vi "Measurement UI.vi"() -> ()   [LabVIEW 2025, in "I2C Bus Monitor UI.lvlib"]
uses:
  I2C Bus Monitor UI.lvlib
  OOB gRPC Client/RPC Messages/hwval_GenericRequest.ctl
  SubVIs/Save CSV.vi
  SubVIs/Table Buffer - Create.vi
  SubVIs/Table Buffer - Destroy.vi
  OOB gRPC Client/OOB gRPC Client.lvlib
panel:
  out "RUNNING":bool
  in  "Monitor Tab":enum32{"Monitor", "Scan"}(tab)
  out "# TXNS IN TABLE":i32
  in  "PauseResume":bool=TRUE
  out "STREAMING":bool
  in  "CSV FILE PATH":path
  in  "Save CSV":bool
  out "# TXNS IN BUFFER":i32
  in  "Clear":bool
  out "MONITOR TABLE":string[][](table)
  in  "Scan Bus":bool
  out "Scan Table":string[][](table)
  out "BUSY":bool
  in  "Debug&Hidden":enum32{"Debug", "Hidden"}(tab)
  out "Message Buffer Pressure (Logic)":i32
  out "Transactions in Buffer (UI)":i32
  out "FIFO Overflow":bool
  out "FIFO Pressure":u32
  out "Measurement Logic Counter":i32
  out "FIFO Msg Fetch Count":i32
  out "OOB gRPC Port":i32
  in  "Bitfile Path":string
  in  "Alias Name":string
  in  "Serial Input":string
  out "Error (Logic)":string
  out "Scanned Addresses":i32[](array[numeric]) format="%.0x"
  out "Status":string
  in  "Send I2C CMD":bool
  in  "R/W":bool
  in  "DATA":u8 format="%02x"
  in  "REG. ADDR.":u16 format="%04x"
  in  "SLAVE ADDR.":u8 format="%02x"
  in  "Send I2C Script":bool
  in  "SCRIPT FILE PATH":path
  in  "SERIAL INPUT (SI)":u32(ring)
  in  "RESOURCE NAME":u32(ring)
  # "NOTE:\nFlat Box sizes are specifically chosen to fit into IS small panel without a horizontal scrollbar"
  # "CONFIGURATION"
  # "I2C TRANSACTIONS"
  # "I2C MONITOR"
  # "STATUS"
  # "These controls are mainly used to transfer data from logic to ui via configs/results, but don't need to be visible."
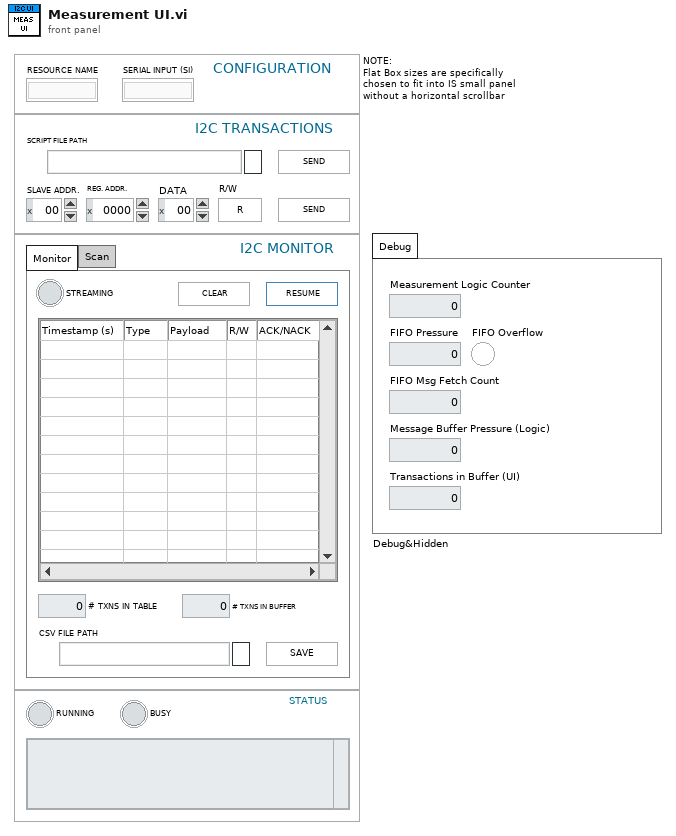
[diagram p1: front panel]
types:
  T1 = cluster{"Measurement Logic Counter":refnum<vi>, "OOB gRPC Port":refnum<vi>, "Bitfile Path":refnum<vi>, "RESOURCE NAME":refnum<vi>, "Alias Name":refnum<vi>, "SERIAL INPUT (SI)":refnum<vi>, "Serial Input":refnum<vi>, "MONITOR TABLE":refnum<vi>, "FIFO Msg Fetch Count":refnum<vi>, "STREAMING":refnum<vi>, "PauseResume":refnum<vi>, "Transactions in Buffer (UI)":refnum<vi>, "CSV FILE PATH":refnum<vi>, "BUSY":refnum<vi>, "Status":refnum<vi>, "Error (Logic)":refnum<vi>, "Scan Table":refnum<vi>, "Scanned Addresses":refnum<vi>, "# TXNS IN BUFFER":refnum<vi>, "# TXNS IN TABLE":refnum<vi>, "RUNNING":refnum<vi>}
  T2 = typedef "OOB gRPC Client.lvlib/hwval_GenericRequest.ctl" = cluster{"Command":string, "Payload":u8[]}
  T3 = typedef "OOB gRPC Client.lvlib/hwval_GenericResponse.ctl" = cluster{"Payload":u8[]}
  T4 = typedef "grpc-lvsupport-release.lvlib/grpcId.ctl" = u64
  T5 = cluster{"NewVal":bool, "SLAVE ADDR.":u8, "REG. ADDR.":u16, "DATA":u8, "R/W":bool}
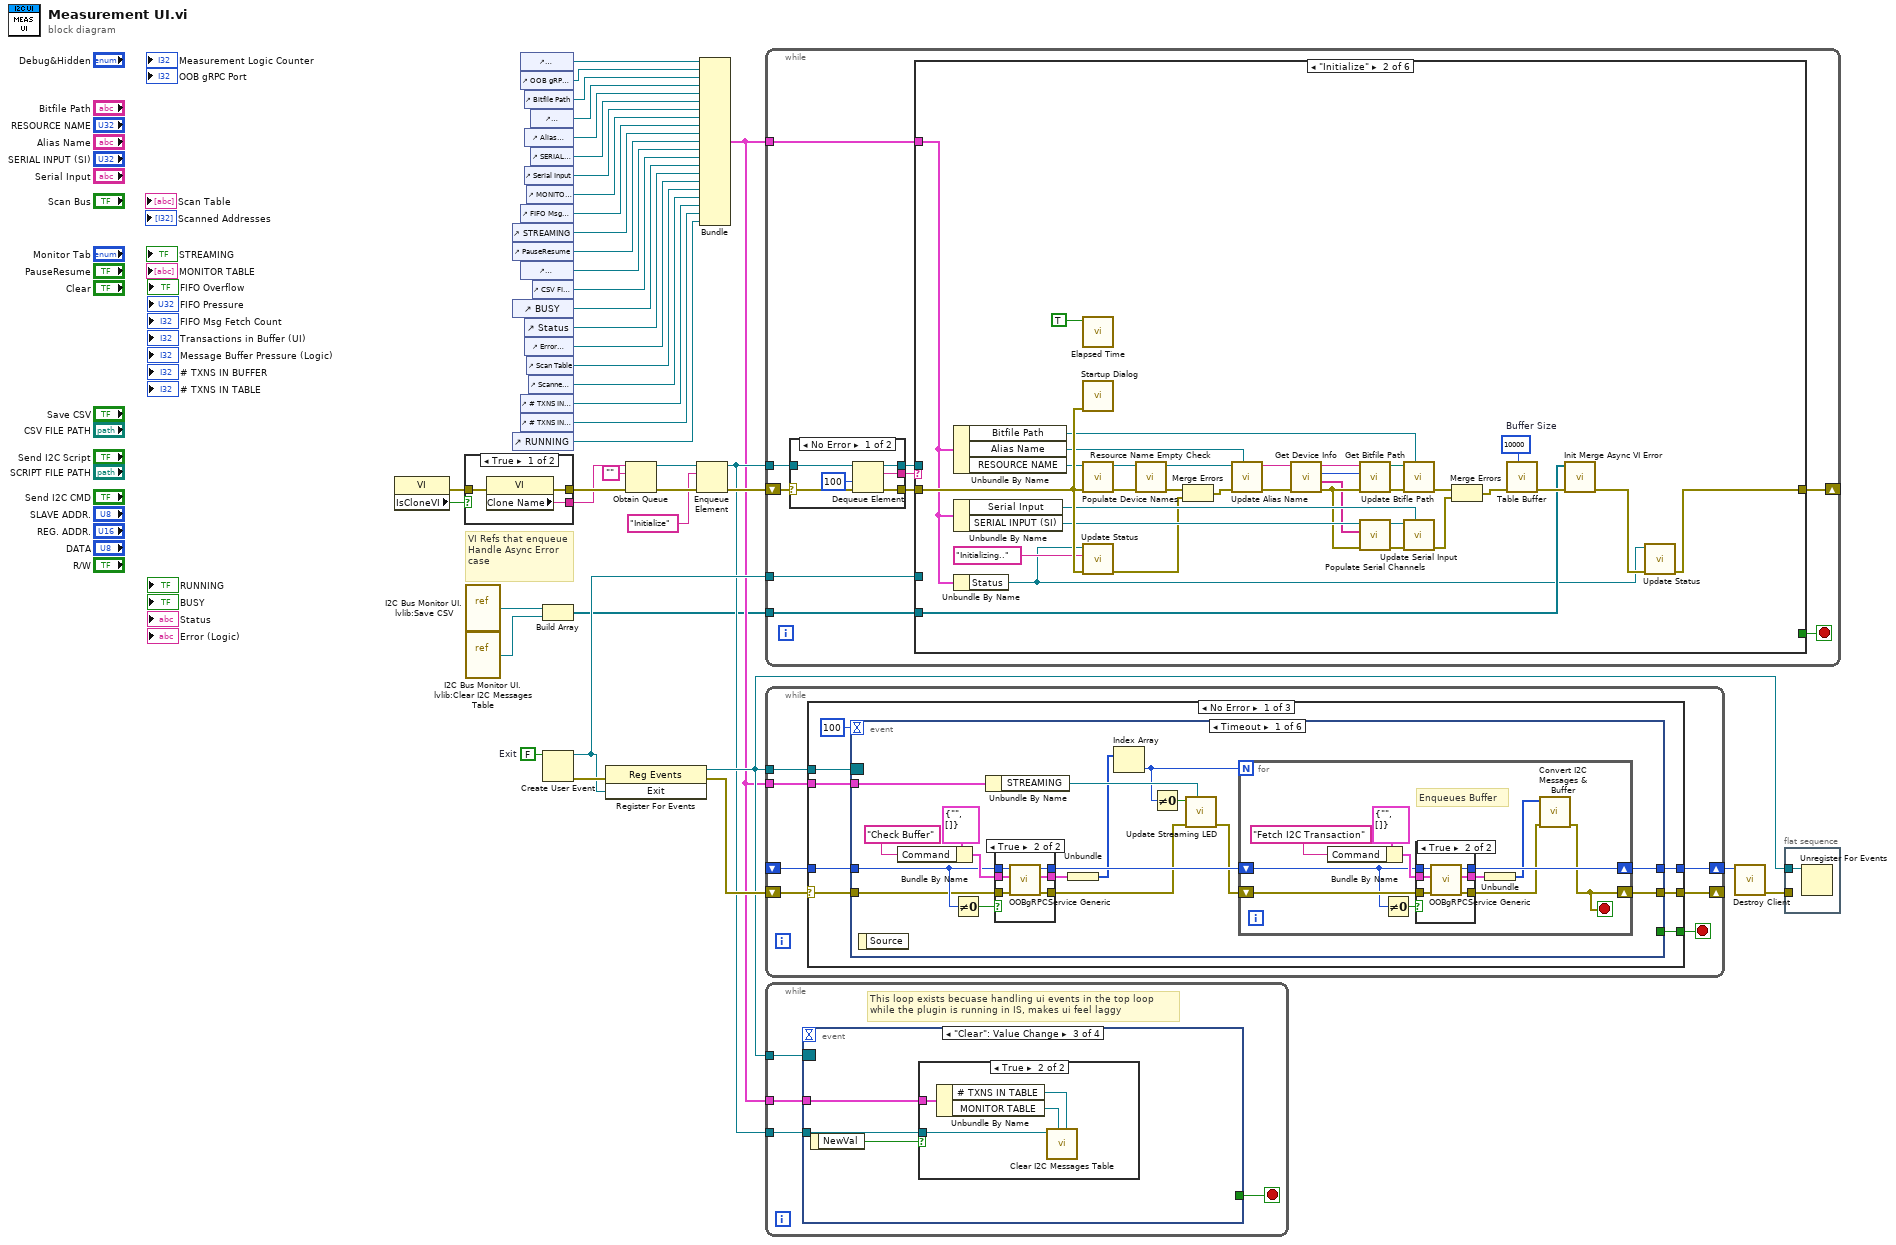
[diagram p0: block diagram]
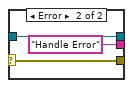
[diagram p2: hidden frame]
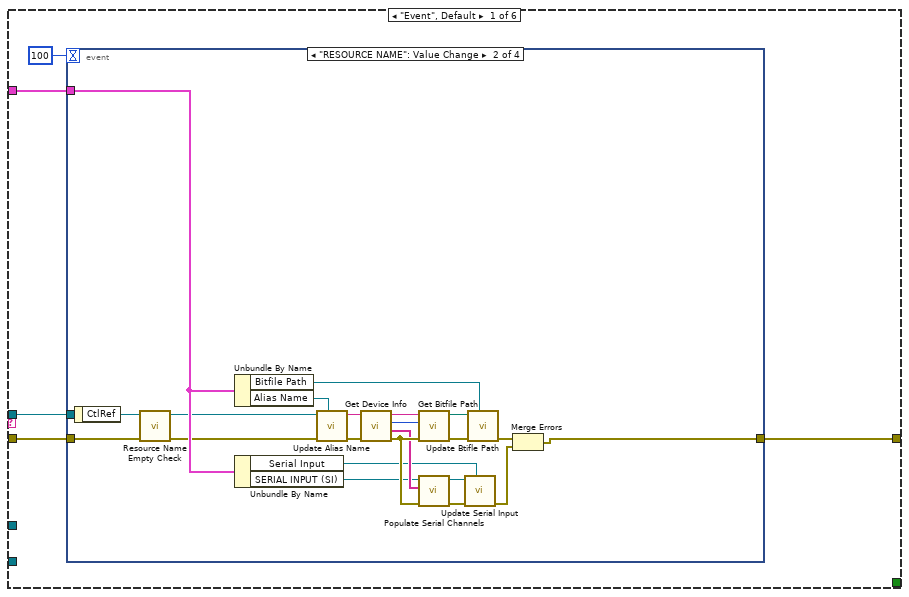
[diagram p3: hidden frame]
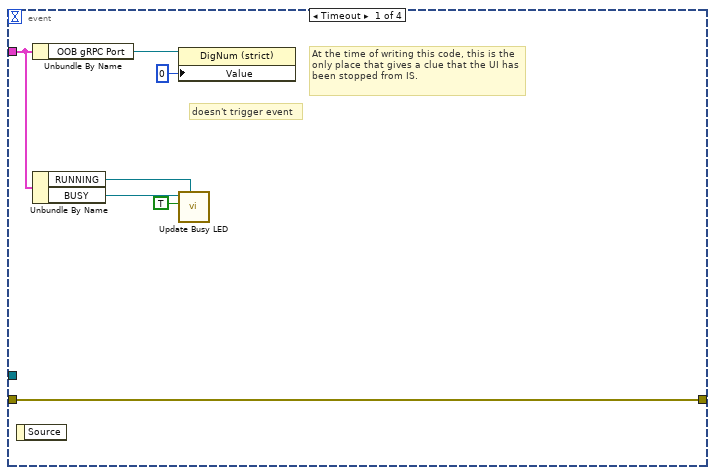
[diagram p4: hidden frame]
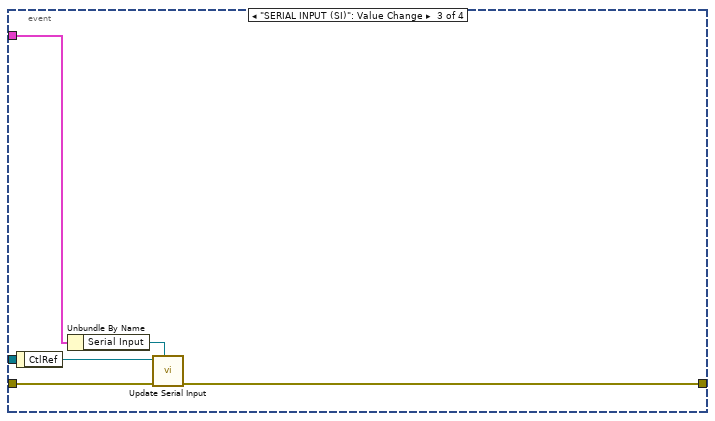
[diagram p5: hidden frame]
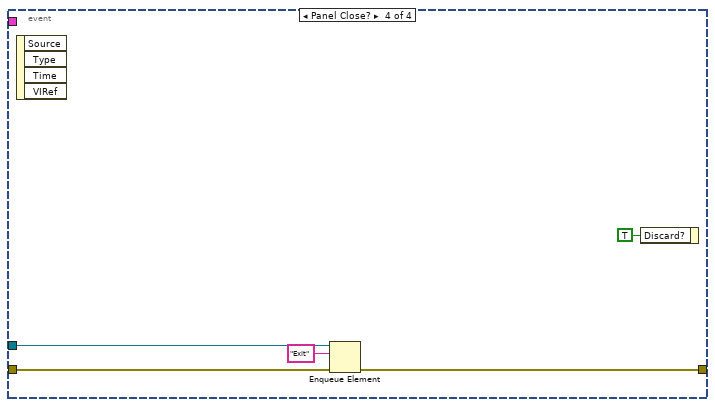
[diagram p6: hidden frame]
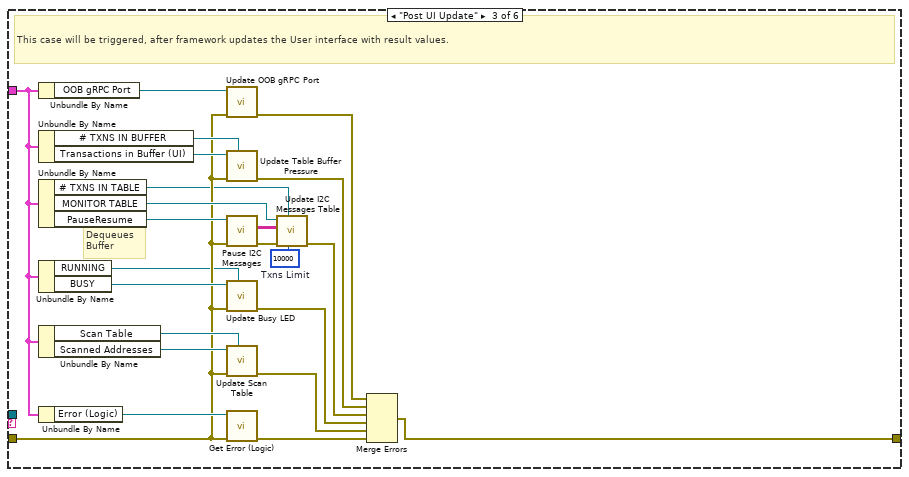
[diagram p7: hidden frame]
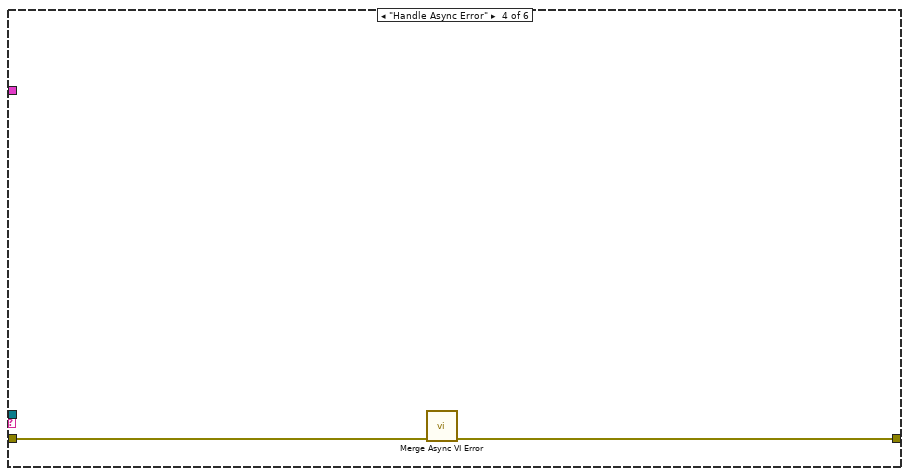
[diagram p8: hidden frame]
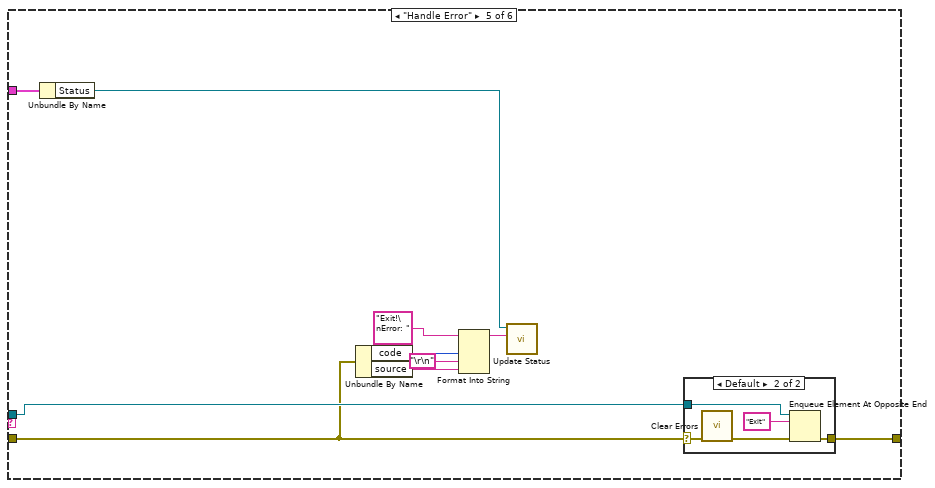
[diagram p9: hidden frame]
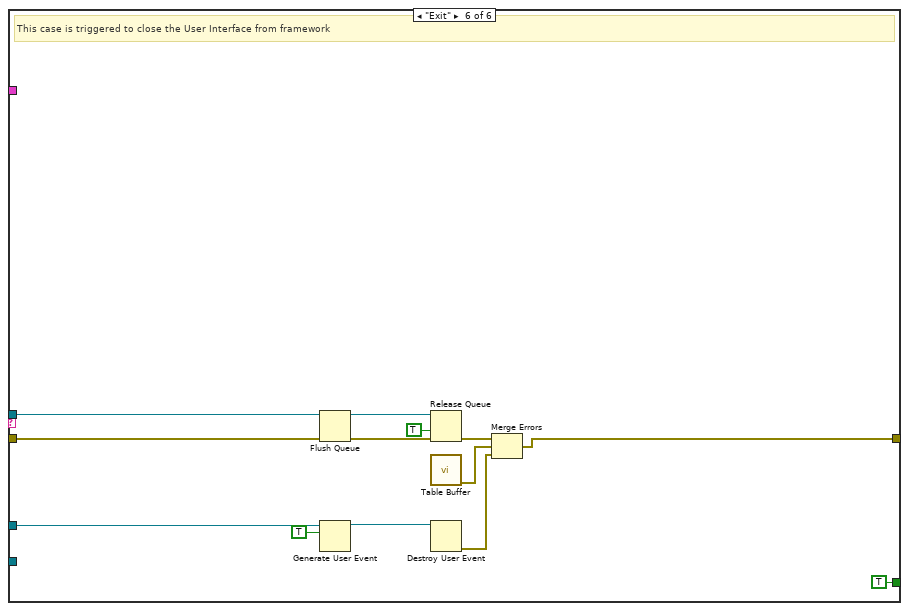
[diagram p11: hidden frame]
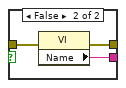
[diagram p12: hidden frame]
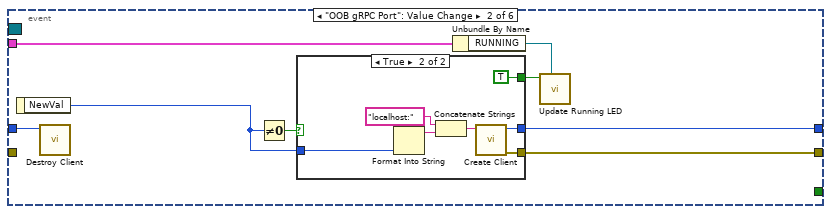
[diagram p15: hidden frame]
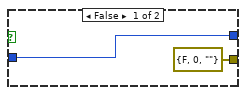
[diagram p16: hidden frame]
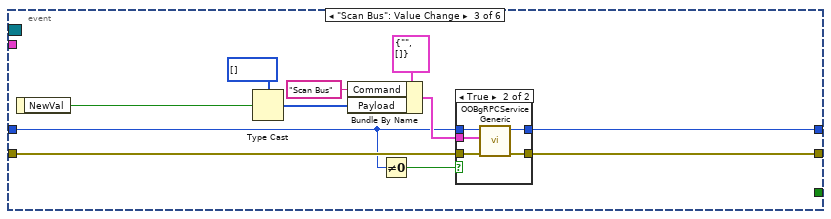
[diagram p17: hidden frame]
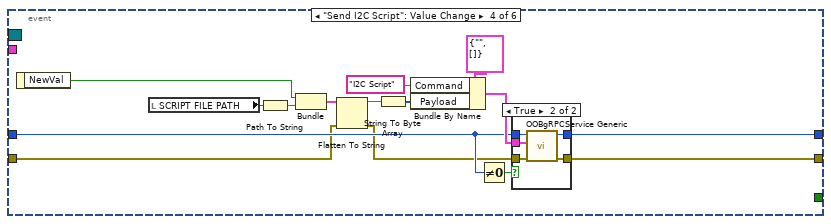
[diagram p19: hidden frame]
diagram:
  w33 = FALSE  # Exit
  # "VI Refs that enqueue Handle Async Error case"
  n1 = property class="VI"() -> (error out=w29:errorcluster, "IsCloneVI"=w34:bool)  [unwired: 2 in, 1 out]
  n2 = case shown="True" w34 {
    tunnel: [w45 w48] -> w41
    tunnel: [w44 w47] -> w40
    tunnel: w29 -> [w43 w46]
    frame True {
      n3 = property class="VI"(error in=w43) -> (error out=w45:errorcluster, "Clone Name"=w44:string)  [unwired: 1 in, 1 out]
    }
    frame False {
      n4 = property class="VI"(error in=w46) -> (error out=w48:errorcluster, "Name"=w47:string)  [unwired: 1 in, 1 out]
    }
  }
  n5 = vi-ref "I2C Bus Monitor UI.lvlib:Save CSV.vi"() -> (w9:refnum<vi>)
  n6 = vi-ref "I2C Bus Monitor UI.lvlib:Clear I2C Messages Table.vi"() -> (w4:refnum<vi>)
  n7 = control-ref of="STREAMING"() -> (w15:refnum<vi>)
  n8 = control-ref of="PauseResume"() -> (w21:refnum<vi>)
  n9 = control-ref of="BUSY"() -> (w13:refnum<vi>)
  n10 = control-ref of="RUNNING"() -> (w1:refnum<vi>)
  n11 = control-ref of="Measurement Logic Counter"() -> (w14:refnum<vi>)
  n12 = control-ref of="OOB gRPC Port"() -> (w27:refnum<vi>)
  n13 = control-ref of="FIFO Msg Fetch Count"() -> (w28:refnum<vi>)
  n14 = control-ref of="Transactions in Buffer (UI)"() -> (w20:refnum<vi>)
  n15 = control-ref of="# TXNS IN BUFFER"() -> (w5:refnum<vi>)
  n16 = control-ref of="# TXNS IN TABLE"() -> (w2:refnum<vi>)
  n17 = control-ref of="Bitfile Path"() -> (w22:refnum<vi>)
  n18 = control-ref of="Alias Name"() -> (w24:refnum<vi>)
  n19 = control-ref of="Serial Input"() -> (w26:refnum<vi>)
  n20 = control-ref of="Status"() -> (w11:refnum<vi>)
  n21 = control-ref of="Error (Logic)"() -> (w10:refnum<vi>)
  n22 = control-ref of="MONITOR TABLE"() -> (w18:refnum<vi>)
  n23 = control-ref of="Scan Table"() -> (w7:refnum<vi>)
  n24 = control-ref of="Scanned Addresses"() -> (w6:refnum<vi>)
  n25 = control-ref of="RESOURCE NAME"() -> (w23:refnum<vi>)
  n26 = control-ref of="SERIAL INPUT (SI)"() -> (w25:refnum<vi>)
  n27 = control-ref of="CSV FILE PATH"() -> (w19:refnum<vi>)
  n28 = Build Array(w9, w4) -> (w8:refnum<vi>[])
  n29 = Create User Event(user event datatype=w33) -> (user event=w30:refnum<user-event>, error out=w32:errorcluster)  [unwired: 1 in]
  n30 = register-events(error in=w32, w30) -> (reference out=w17:refnum<event-registration>, error out=w42:errorcluster)  [unwired: 1 in]
  n31 = Obtain Queue(name (unnamed)=w40, element data type="", error in (no error)=w41) -> (queue out=w37:refnum<queue>, error out=w39:errorcluster)  [unwired: 2 in, 1 out]
  n32 = Enqueue Element(queue=w37, element="Initialize", error in (no error)=w39) -> (queue out=w16:refnum<queue>, error out=w38:errorcluster)  [unwired: 1 in, 1 out]
  n33 = Bundle("Measurement Logic Counter"=w14, "OOB gRPC Port"=w27, "Bitfile Path"=w22, "RESOURCE NAME"=w23, "Alias Name"=w24, "SERIAL INPUT (SI)"=w25, "Serial Input"=w26, "MONITOR TABLE"=w18, "FIFO Msg Fetch Count"=w28, "STREAMING"=w15, "PauseResume"=w21, "Transactions in Buffer (UI)"=w20, "CSV FILE PATH"=w19, "BUSY"=w13, "Status"=w11, "Error (Logic)"=w10, "Scan Table"=w7, "Scanned Addresses"=w6, "# TXNS IN BUFFER"=w5, "# TXNS IN TABLE"=w2, "RUNNING"=w1) -> (w12:T1)  [unwired: 1 in]
  n34 = while {
    shift-right: [w53] -> _
    shift-left: w38 -> [w58]
    tunnel: w16 -> [w56]
    tunnel: w30 -> [w51]
    tunnel: w12 -> [w50]
    tunnel: w8 -> [w49]
    stop <- w52 stop-if-true
    n35 = case shown="No Error" w58 {
      selector: w58 -> [w64 w67]
      tunnel: [w63 w67] -> w57
      tunnel: w56 -> [w62 w66]
      tunnel: [w61 w66] -> w55
      tunnel: [w60 "Handle Error"] -> w54
      frame No Error {
        n36 = Dequeue Element(queue=w62, timeout in ms (-1)=100, error in (no error)=w64) -> (queue out=w61:refnum<queue>, element=w60:string, error out=w63:errorcluster)  [unwired: 1 out]
      }
      frame Error {
      }
    }
    n37 = case shown="\"Initialize\"" w54 {
      tunnel: w57 -> [w71 w145 w149 w170 w175 w190]
      tunnel: w55 -> [w69 _ _ _ w176 w198]
      tunnel: [w72 w113 w167 w169 w174 w189] -> w53
      tunnel: [_ _ _ _ _ TRUE] -> w52
      tunnel: w51 -> [_ _ _ _ _ w191]
      tunnel: w50 -> [w68 w135 w155 _ w172 _]
      tunnel: w49 -> [_ w137 _ _ _ _]
      frame "Event", Default {
        n38 = event shown="[1] \"RESOURCE NAME\": Value Change" {
          selector: _ -> [_ _ _ _]
          dyn-events: _ -> [_ _ _ _]
          timeout: 100 -> [_ _ _ _]
          tunnel: [w79 w96 w102 w109] -> w72
          tunnel: w71 -> [w79 w92 w106 w110]
          tunnel: w69 -> [_ _ _ w108]
          tunnel: w68 -> [w76 w94 w104 _]
          event Timeout {
            # "doesn't trigger event"
            # "At the time of writing this code, this is the only place that gives a clue that the UI has been stopped from IS."
            n39 = event-data() -> ()  [unwired: 1 in, 1 out]
            n40 = Unbundle By Name(w76) -> ("OOB gRPC Port"=w77:refnum<vi>)
            n41 = Unbundle By Name(w76) -> ("RUNNING"=w73:refnum<vi>, "BUSY"=w74:refnum<vi>)
            n42 = property on="Property Node" class="DigNum (strict)"(reference=w77, "Value"=0 ("OOB gRPC Port")) -> ()  [unwired: 1 in, 2 out]
            n43 = call "Update Busy LED.vi"("RUNNING Ref"=w73, "Busy (False)"=TRUE ("value"), "BUSY Ref"=w74) -> ()  [unwired: 8 in, 1 out]
          }
          event "RESOURCE NAME": Value Change {
            n44 = event-data() -> ("CtlRef"=w81:refnum<vi>)  [unwired: 1 in]
            n45 = call "Resource Name Empty Check.vi"("error in (no error)"=w92, "RESOURCE NAME Ref"=w81) -> ("error out"=w82:errorcluster, "RESOURCE NAME Ref out"=w80:refnum<vi>)  [unwired: 8 in]
            n46 = Unbundle By Name(w94) -> ("Bitfile Path"=w84:refnum<vi>, "Alias Name"=w89:refnum<vi>)
            n47 = Unbundle By Name(w94) -> ("Serial Input"=w86:refnum<vi>, "SERIAL INPUT (SI)"=w93:refnum<vi>)
            n48 = call "Update Alias Name.vi"("Alias Name Ref"=w89, "error in (no error)"=w82, "RESOURCE NAME Ref"=w80) -> ("error out"=w90:errorcluster, "Alias Name"=w91:string)  [unwired: 7 in]
            n49 = call "Get Device Info.vi"("error in (no error)"=w90, "RIO Device"=w91) -> ("error out"=w101:errorcluster, "SI Channels"=w98:string[], "SI Count"=w100:i32, "Module Name"=w99:string)  [unwired: 6 in]
            n50 = call "Get Bitfile Path.vi"("error in (no error)"=w101, "SI Count"=w100, "Module Name"=w99) -> ("error out"=w97:errorcluster, "Bitfile Path"=w83:path)  [unwired: 7 in]
            n51 = call "Populate Serial Channels.vi"("error in (no error)"=w101, "Strings []"=w98, "SERIAL INPUT (SI) Ref in"=w93) -> ("error out"=w95:errorcluster, "SERIAL INPUT (SI) Ref out"=w87:refnum<vi>)  [unwired: 7 in]
            n52 = call "Update Serial Input.vi"("Serial Input Ref"=w86, "error in (no error)"=w95, "SERIAL INPUT (SI) Ref"=w87) -> ("error out"=w88:errorcluster)  [unwired: 8 in]
            n53 = call "Update Btifle Path.vi"("Bitfile Path Ref"=w84, "error in (no error)"=w97, "Bitfile Path"=w83) -> ("error out"=w85:errorcluster)  [unwired: 8 in]
            n54 = Merge Errors(w85, w88) -> (w96:errorcluster)
          }
          event "SERIAL INPUT (SI)": Value Change {
            n55 = event-data() -> ("CtlRef"=w105:refnum<vi>)  [unwired: 1 in]
            n56 = Unbundle By Name(w104) -> ("Serial Input"=w103:refnum<vi>)
            n57 = call "Update Serial Input.vi"("Serial Input Ref"=w103, "error in (no error)"=w106, "SERIAL INPUT (SI) Ref"=w105) -> ("error out"=w102:errorcluster)  [unwired: 8 in]
          }
          event Panel Close? {
            n58 = event-data() -> ()  [unwired: 1 in, 4 out]
            n59 = Enqueue Element(queue=w108, element="Exit", error in (no error)=w110) -> (error out=w109:errorcluster)  [unwired: 1 in, 2 out]
            n60 = event-data("Discard?"=TRUE) -> ()  [unwired: 1 in, 1 out]
          }
        }
      }
      frame "Initialize" {
        w136 = 10000  # Buffer Size
        n61 = Unbundle By Name(w135) -> ("Bitfile Path"=w140:refnum<vi>, "Alias Name"=w142:refnum<vi>, "RESOURCE NAME"=w144:refnum<vi>)
        n62 = Unbundle By Name(w135) -> ("Serial Input"=w141:refnum<vi>, "SERIAL INPUT (SI)"=w143:refnum<vi>)
        n63 = Unbundle By Name(w135) -> ("Status"=w112:refnum<vi>)
        n64 = call "Elapsed Time.vi"("Reset"=TRUE) -> ()  [unwired: 9 in, 2 out]
        n65 = call "Startup Dialog.vi"("error in"=w145) -> ()  [unwired: 10 in, 1 out]
        n66 = call "Populate Device Names.vi"("error in (no error)"=w145, "RESOURCE NAME Ref"=w144) -> ("error out"=w116:errorcluster, "RESOURCE NAME Ref out"=w133:refnum<vi>)  [unwired: 8 in]
        n67 = call "Update Status.vi"("error in (no error)"=w145, "Value"="Initializing..", "Status Ref"=w112) -> ("error out"=w129:errorcluster)  [unwired: 8 in]
        n68 = call "Resource Name Empty Check.vi"("error in (no error)"=w116, "RESOURCE NAME Ref"=w133) -> ("error out"=w115:errorcluster, "RESOURCE NAME Ref out"=w132:refnum<vi>)  [unwired: 8 in]
        n69 = Merge Errors(w115, w129) -> (w131:errorcluster)
        n70 = call "Update Alias Name.vi"("Alias Name Ref"=w142, "error in (no error)"=w131, "RESOURCE NAME Ref"=w132) -> ("error out"=w122:errorcluster, "Alias Name"=w121:string)  [unwired: 7 in]
        n71 = call "Get Device Info.vi"("error in (no error)"=w122, "RIO Device"=w121) -> ("error out"=w128:errorcluster, "SI Channels"=w125:string[], "SI Count"=w127:i32, "Module Name"=w126:string)  [unwired: 6 in]
        n72 = call "Get Bitfile Path.vi"("error in (no error)"=w128, "SI Count"=w127, "Module Name"=w126) -> ("error out"=w124:errorcluster, "Bitfile Path"=w117:path)  [unwired: 7 in]
        n73 = call "Populate Serial Channels.vi"("error in (no error)"=w128, "Strings []"=w125, "SERIAL INPUT (SI) Ref in"=w143) -> ("error out"=w123:errorcluster, "SERIAL INPUT (SI) Ref out"=w119:refnum<vi>)  [unwired: 7 in]
        n74 = call "Update Btifle Path.vi"("Bitfile Path Ref"=w140, "error in (no error)"=w124, "Bitfile Path"=w117) -> ("error out"=w118:errorcluster)  [unwired: 8 in]
        n75 = call "Update Serial Input.vi"("Serial Input Ref"=w141, "error in (no error)"=w123, "SERIAL INPUT (SI) Ref"=w119) -> ("error out"=w120:errorcluster)  [unwired: 8 in]
        n76 = Merge Errors(w118, w120) -> (w130:errorcluster)
        n77 = call-poly "Table Buffer.vi"("Buffer Size (10k)"=w136, "error in (no error)"=w130) -> ("error out"=w139:errorcluster)  [unwired: 9 in]
        n78 = call "Init Merge Async VI Error.vi"("error in (no error)"=w139, "VI Ref"=w137) -> ("error out"=w114:errorcluster)  [unwired: 9 in]
        n79 = call "Update Status.vi"("error in (no error)"=w114, "Status Ref"=w112) -> ("error out"=w113:errorcluster)  [unwired: 9 in]
      }
      frame "Post UI Update" {
        w147 = 10000  # Txns Limit
        # "Dequeues Buffer"
        # "This case will be triggered, after framework updates the User interface with result values."
        n80 = Unbundle By Name(w155) -> ("OOB gRPC Port"=w168:refnum<vi>)
        n81 = Unbundle By Name(w155) -> ("# TXNS IN BUFFER"=w152:refnum<vi>, "Transactions in Buffer (UI)"=w160:refnum<vi>)
        n82 = Unbundle By Name(w155) -> ("# TXNS IN TABLE"=w148:refnum<vi>, "MONITOR TABLE"=w162:refnum<vi>, "PauseResume"=w161:refnum<vi>)
        n83 = Unbundle By Name(w155) -> ("RUNNING"=w146:refnum<vi>, "BUSY"=w157:refnum<vi>)
        n84 = Unbundle By Name(w155) -> ("Scan Table"=w154:refnum<vi>, "Scanned Addresses"=w153:refnum<vi>)
        n85 = Unbundle By Name(w155) -> ("Error (Logic)"=w156:refnum<vi>)
        n86 = call "Update OOB gRPC Port.vi"("error in (no error)"=w149, "OOB gRPC Port Ref in"=w168) -> ("error out"=w166:errorcluster)  [unwired: 9 in]
        n87 = call "Update Table Buffer Pressure.vi"("BUFFER Ref"=w152, "error in (no error)"=w149, "Table Buffer Pressure Ref"=w160) -> ("error out"=w159:errorcluster)  [unwired: 8 in]
        n88 = call "Pause I2C Messages.vi"("error in (no error)"=w149, "PauseResume Ref"=w161) -> ("error out"=w164:errorcluster, "I2C Messages"=w163:string[][])  [unwired: 8 in]
        n89 = call "Update Busy LED.vi"("RUNNING Ref"=w146, "error in (no error)"=w149, "BUSY Ref"=w157) -> ("error out"=w158:errorcluster)  [unwired: 8 in]
        n90 = call "Update Scan Table.vi"("Scan Table Ref"=w154, "error in (no error)"=w149, "Scanned Addresses Ref"=w153) -> ("error out"=w150:errorcluster)  [unwired: 8 in]
        n91 = call "Get Error (Logic).vi"("error in (no error)"=w149, "Error (Logic)Ref"=w156) -> ("error out"=w151:errorcluster)  [unwired: 9 in]
        n92 = call "Update I2C Messages Table.vi"("Transactions Limit (10k)"=w147, "# TXNS IN TABLE Ref"=w148, "error in (no error)"=w164, "I2C Messages in"=w163, "I2C Table Ref"=w162) -> ("error out"=w165:errorcluster)  [unwired: 6 in]
        n93 = Merge Errors(w166, w159, w165, w158, w150, w151) -> (w167:errorcluster)
      }
      frame "Handle Async Error" {
        n94 = call "Merge Async VI Error.vi"("error in (no error)"=w170) -> ("error out"=w169:errorcluster)  [unwired: 10 in]
      }
      frame "Handle Error" {
        n95 = Unbundle By Name(w172) -> ("Status"=w173:refnum<vi>)
        n96 = Unbundle By Name(w175) -> ("code"=w180:i32, "source"=w179:string)
        n97 = Format Into String(initial string="Exit!\nError: " ("format string"), w180, "\r\n", w179) -> (resulting string=w171:string)  [unwired: 2 in, 1 out]
        n98 = call "Update Status.vi"("Value"=w171, "Status Ref"=w173) -> ()  [unwired: 9 in, 1 out]
        n99 = case shown="Default" w175 {
          selector: w175 -> [w181 w186]
          tunnel: [w181 w185] -> w174
          tunnel: w176 -> [_ w183]
          frame No Error {
          }
          frame Default {
            n100 = call <vilib>:"Clear Errors.vi"("error in (no error)"=w186) -> ("error out"=w184:errorcluster)  [unwired: 5 in, 1 out]
            n101 = Enqueue Element At Opposite End(queue=w183, element="Exit", error in (no error)=w184) -> (error out=w185:errorcluster)  [unwired: 1 in, 2 out]
          }
        }
      }
      frame "Exit" {
        # "This case is triggered to close the User Interface from framework"
        n102 = Flush Queue(queue=w198, error in (no error)=w190) -> (queue out=w197:refnum<queue>, error out=w196:errorcluster)  [unwired: 1 out]
        n103 = Generate User Event(user event=w191, event data cluster=TRUE ("event data")) -> (user event out=w192:refnum<user-event>)  [unwired: 2 in, 1 out]
        n104 = Release Queue(queue=w197, force destroy? (F)=TRUE, error in (no error)=w196) -> (error out=w195:errorcluster)  [unwired: 2 out]
        n105 = call-poly "Table Buffer.vi"() -> ("error out"=w187:errorcluster)  [unwired: 11 in]
        n106 = Destroy User Event(user event=w192) -> (error out=w188:errorcluster)  [unwired: 1 in]
        n107 = Merge Errors(w195, w187, w188) -> (w189:errorcluster)
      }
    }
  }
  n108 = while {
    tunnel: w17 -> [w203]
    shift-right: [w204] -> _
    shift-left: w42 -> [w206]
    shift-right: [w201] -> w31
    shift-left: _ -> [w202]
    tunnel: w12 -> [w200]
    stop <- w205 stop-if-true
    n109 = case shown="No Error" w206 {
      selector: w206 -> [w212 w343 _]
      tunnel: [w209 TRUE w353] -> w205
      tunnel: [w213 w343 errorcluster {"status"=FALSE, "code"=0, "source"=""} ("error IO")] -> w204
      tunnel: w203 -> [w214 _ _]
      tunnel: w202 -> [w211 w344 w352]
      tunnel: [w210 w344 w352] -> w201
      tunnel: w200 -> [w207 _ w347]
      frame No Error {
        n110 = event shown="[0] Timeout" {
          selector: w214 -> [_ _ _ _ _ _]
          dyn-events: _ -> [_ _ _ _ _ _]
          timeout: 100 -> [_ _ _ _ _ _]
          tunnel: [w229 w266 w279 w303 w327 w340] -> w213
          tunnel: w212 -> [w222 _ w278 w295 w321 w340]
          tunnel: w211 -> [w223 w265 w277 w302 w326 w341]
          tunnel: [w230 w264 w280 w304 w328 w341] -> w210
          tunnel: [_ _ _ _ _ w342] -> w209
          tunnel: w207 -> [w219 w261 _ _ _ _]
          event Timeout {
            n111 = event-data() -> ()  [unwired: 1 in, 1 out]
            n112 = Bundle By Name(cluster=T2 {"Command"="", "Payload"=[]} ("Request Data"), "Command"="Check Buffer") -> (w226:T2)
            n113 = Not Equal To 0?(x=w223) -> (x != 0?=w225:bool)
            n114 = Unbundle By Name(w219) -> ("STREAMING"=w231:refnum<vi>)
            n115 = case shown="True" w225 {
              tunnel: [w252 w255] -> w221
              tunnel: [w251 w254] -> w218
              tunnel: w223 -> [w252 w258]
              tunnel: w222 -> [w251 w257]
              tunnel: w226 -> [_ w256]
              tunnel: [_ w253] -> w228
              frame False {
              }
              frame True {
                n116 = call "OOBgRPCService Generic.vi"("error in"=w257, "Request Data"=w256, "gRPC ID"=w258) -> ("error out"=w254:errorcluster, "Response Data"=w253:T3, "gRPC ID out"=w255:T4)  [unwired: 6 in]
              }
            }
            n117 = Unbundle(w228) -> ("Payload"=w220:u8[])
            n118 = Index Array(array=w220) -> (element=w215:u8)  [unwired: 1 in]
            n119 = Not Equal To 0?(x=w215) -> (x != 0?=w216:bool)
            n120 = call "Update Streaming LED.vi"("STREAMING Ref"=w231, "error in (no error)"=w218, "Value"=w216) -> ("error out"=w217:errorcluster)  [unwired: 8 in]
            n121 = for {
              N: w215 -> [_]
              shift-right: [w233] -> w229
              shift-left: w217 -> [w242]
              shift-right: [w237] -> w230
              shift-left: w221 -> [w234]
              stop <- w233 stop-if-true
              # "Enqueues Buffer"
              n122 = Bundle By Name(cluster=T2 {"Command"="", "Payload"=[]} ("Request Data"), "Command"="Fetch I2C Transaction") -> (w240:T2)
              n123 = Not Equal To 0?(x=w234) -> (x != 0?=w241:bool)
              n124 = case shown="True" w241 {
                tunnel: [w244 w247] -> w237
                tunnel: [w243 w246] -> w235
                tunnel: w234 -> [w244 w250]
                tunnel: w242 -> [w243 w249]
                tunnel: w240 -> [_ w248]
                tunnel: [_ w245] -> w236
                frame False {
                }
                frame True {
                  n125 = call "OOBgRPCService Generic.vi"("error in"=w249, "Request Data"=w248, "gRPC ID"=w250) -> ("error out"=w246:errorcluster, "Response Data"=w245:T3, "gRPC ID out"=w247:T4)  [unwired: 6 in]
                }
              }
              n126 = Unbundle(w236) -> ("Payload"=w232:u8[])
              n127 = call "Convert I2C Messages & Buffer.vi"("error in (no error)"=w235, "Data"=w232) -> ("error out"=w233:errorcluster)  [unwired: 9 in]
            }
          }
          event "OOB gRPC Port": Value Change {
            n128 = event-data() -> ("NewVal"=w262:i32)  [unwired: 1 in]
            n129 = call "Destroy Client.vi"("gRPC ID"=w265) -> ()  [unwired: 10 in, 1 out]
            n130 = Not Equal To 0?(x=w262) -> (x != 0?=w263:bool)
            n131 = case shown="True" w263 {
              tunnel: [errorcluster {"status"=FALSE, "code"=0, "source"=""} ("error out") w275] -> w266
              tunnel: w262 -> [w268 w271]
              tunnel: [w268 w270] -> w264
              tunnel: [_ TRUE ("Value")] -> w259
              frame False {
              }
              frame True {
                n132 = Format Into String(w271) -> (resulting string=w274:string)  [unwired: 3 in, 1 out]
                n133 = Concatenate Strings("localhost:" ("string"), w274) -> (w272:string)
                n134 = call "Create Client.vi"("address"=w272) -> ("error out"=w275:errorcluster, "gRPC ID Out"=w270:T4)  [unwired: 9 in]
              }
            }
            n135 = Unbundle By Name(w261) -> ("RUNNING"=w260:refnum<vi>)
            n136 = call "Update Running LED.vi"("RUNNING Ref"=w260, "Value"=w259) -> ()  [unwired: 9 in, 1 out]
          }
          event "Scan Bus": Value Change {
            n137 = event-data() -> ("NewVal"=w276:bool)  [unwired: 1 in]
            n138 = Type Cast(type=u8[] [] ("Payload"), x=w276) -> (*(type *) &x=w286:u8[])
            n139 = Bundle By Name(cluster=T2 {"Command"="", "Payload"=[]} ("Request Data"), "Command"="Scan Bus", "Payload"=w286) -> (w284:T2)
            n140 = Not Equal To 0?(x=w277) -> (x != 0?=w285:bool)
            n141 = case shown="True" w285 {
              tunnel: [w288 w290] -> w280
              tunnel: [w287 w289] -> w279
              tunnel: w277 -> [w288 w293]
              tunnel: w278 -> [w287 w292]
              tunnel: w284 -> [_ w291]
              frame False {
              }
              frame True {
                n142 = call "OOBgRPCService Generic.vi"("error in"=w292, "Request Data"=w291, "gRPC ID"=w293) -> ("error out"=w289:errorcluster, "gRPC ID out"=w290:T4)  [unwired: 6 in, 1 out]
              }
            }
          }
          event "Send I2C Script": Value Change {
            n143 = event-data() -> ("NewVal"=w299:bool)  [unwired: 1 in]
            n144 = local read "SCRIPT FILE PATH"() -> (w300:path)
            n145 = Path To String(path=w300) -> (string=w301:string)
            n146 = Bundle("NewVal"=w299, w301) -> (w298:cluster{"NewVal":bool, string})  [unwired: 1 in]
            n147 = Flatten To String(anything=w298, error in (no error)=w295) -> (data string=w297:string, error out=w294:errorcluster)  [unwired: 2 in, 1 out]
            n148 = String To Byte Array(string=w297) -> (unsigned byte array=w296:u8[])
            n149 = Bundle By Name(cluster=T2 {"Command"="", "Payload"=[]} ("Request Data"), "Command"="I2C Script", "Payload"=w296) -> (w307:T2)
            n150 = Not Equal To 0?(x=w302) -> (x != 0?=w308:bool)
            n151 = case shown="True" w308 {
              tunnel: [w310 w312] -> w304
              tunnel: [w309 w311] -> w303
              tunnel: w302 -> [w310 w315]
              tunnel: w294 -> [w309 w314]
              tunnel: w307 -> [_ w313]
              frame False {
              }
              frame True {
                n152 = call "OOBgRPCService Generic.vi"("error in"=w314, "Request Data"=w313, "gRPC ID"=w315) -> ("error out"=w311:errorcluster, "gRPC ID out"=w312:T4)  [unwired: 6 in, 1 out]
              }
            }
          }
          event "Send I2C CMD": Value Change {
            n153 = event-data() -> ("NewVal"=w325:bool)  [unwired: 1 in]
            n154 = local read "SLAVE ADDR."() -> (w319:u8)
            n155 = local read "REG. ADDR."() -> (w318:u16)
            n156 = local read "DATA"() -> (w317:u8)
            n157 = local read "R/W"() -> (w316:bool)
            n158 = Bundle("NewVal"=w325, "SLAVE ADDR."=w319, "REG. ADDR."=w318, "DATA"=w317, "R/W"=w316) -> (w324:T5)  [unwired: 1 in]
            n159 = Flatten To String(anything=w324, error in (no error)=w321) -> (data string=w323:string, error out=w320:errorcluster)  [unwired: 2 in, 1 out]
            n160 = String To Byte Array(string=w323) -> (unsigned byte array=w322:u8[])
            n161 = Bundle By Name(cluster=T2 {"Command"="", "Payload"=[]} ("Request Data"), "Command"="I2C CMD", "Payload"=w322) -> (w331:T2)
            n162 = Not Equal To 0?(x=w326) -> (x != 0?=w332:bool)
            n163 = case shown="True" w332 {
              tunnel: [w334 w336] -> w328
              tunnel: [w333 w335] -> w327
              tunnel: w326 -> [w334 w339]
              tunnel: w320 -> [w333 w338]
              tunnel: w331 -> [_ w337]
              frame False {
              }
              frame True {
                n164 = call "OOBgRPCService Generic.vi"("error in"=w338, "Request Data"=w337, "gRPC ID"=w339) -> ("error out"=w335:errorcluster, "gRPC ID out"=w336:T4)  [unwired: 6 in, 1 out]
              }
            }
          }
          event User Event {
            n165 = event-data() -> ("Exit"=w342:bool)  [unwired: 1 in]
          }
        }
      }
      frame Default {
      }
      frame Error {
        n166 = Unbundle By Name(w347) -> ("Status"=w350:refnum<vi>)
        n167 = Unbundle By Name(w347) -> ("RUNNING"=w348:refnum<vi>)
        n168 = local read "OOB gRPC Port"() -> (w355:i32)
        n169 = call "Update Running LED.vi"("RUNNING Ref"=w348, "Value"=FALSE) -> ()  [unwired: 9 in, 1 out]
        n170 = Equal?(x=w355, y=-1 ("x")) -> (x = y?=w353:bool)
        n171 = case shown="False" w353 {
          tunnel: w355 -> [w357 _]
          tunnel: [w356 "OOB gRPC server side Error.\nMeasrement Logic didn't get the gRPC port from OOB server.\nRestart the plugin." ("Status")] -> w349
          frame False {
            # "triggers event"
            n172 = disable-structure shown="Enabled" {
              disable-tunnel: ["OOB gRPC Disconnted!\nReconnecting.." ("Status") _] -> w356
              frame Disabled {
              }
              frame Enabled {
              }
            }
            n173 = property on="OOB gRPC Port" class="DigNum (strict)"("Val(Sgnl)"=w357) -> ()  [unwired: 2 in, 2 out]
          }
          frame True {
          }
        }
        n174 = call "Update Status.vi"("Value"=w349, "Status Ref"=w350) -> ()  [unwired: 9 in, 1 out]
      }
    }
  }
  n175 = while {
    tunnel: w17 -> [w362]
    tunnel: w12 -> [w361]
    tunnel: w16 -> [w360]
    stop <- w363 stop-if-true
    # "This loop exists becuase handling ui events in the top loop while the plugin is running in IS, makes ui feel laggy"
    n176 = event shown="[2] \"Clear\": Value Change" {
      selector: w362 -> [_ _ _ _]
      dyn-events: _ -> [_ _ _ _]
      timeout: _ -> [_ _ _ _]
      tunnel: [_ _ _ w378] -> w363
      tunnel: w361 -> [_ w366 w373 _]
      tunnel: w360 -> [_ w365 w372 _]
      event Timeout {
        n177 = event-data() -> ()  [unwired: 1 in, 1 out]
      }
      event "Save CSV": Value Change {
        n178 = event-data() -> ("NewVal"=w364:bool)  [unwired: 1 in]
        n179 = case shown="True" w364 {
          tunnel: w366 -> [_ w368]
          tunnel: w365 -> [_ w367]
          frame False {
          }
          frame True {
            n180 = Unbundle By Name(w368) -> ("CSV FILE PATH"=w370:refnum<vi>, "MONITOR TABLE"=w369:refnum<vi>)
            n181 = call "Save CSV (Async).vi"("CSV File Ref"=w370, "MONITOR TABLE Ref"=w369, "Measurement UI Queue"=w367) -> ()  [unwired: 8 in, 1 out]
          }
        }
      }
      event "Clear": Value Change {
        n182 = event-data() -> ("NewVal"=w371:bool)  [unwired: 1 in]
        n183 = case shown="True" w371 {
          tunnel: w373 -> [_ w377]
          tunnel: w372 -> [_ w375]
          frame False {
          }
          frame True {
            n184 = Unbundle By Name(w377) -> ("# TXNS IN TABLE"=w374:refnum<vi>, "MONITOR TABLE"=w376:refnum<vi>)
            n185 = call "Clear I2C Messages Table.vi"("# TXNS IN TABLE Ref"=w374, "I2C Table Ref"=w376, "Measurement UI Queue"=w375) -> ()  [unwired: 8 in, 1 out]
          }
        }
      }
      event User Event {
        n186 = event-data() -> ("Exit"=w378:bool)  [unwired: 1 in]
      }
    }
  }
  n187 = call "Destroy Client.vi"("gRPC ID"=w31) -> ("error out"=w3:errorcluster)  [unwired: 10 in]
  n188 = flat-sequence {
    tunnel: w17 -> [w379]
    tunnel: w3 -> [_]
    frame #0 {
      n189 = Unregister For Events(event registration refnum=w379) -> ()  [unwired: 1 in, 1 out]
    }
  }
